vi "dsfsdfsd_Static1.vi"(8 "error in (no error)":errorcluster, 11 "dsfsdfsd in 1":refnum<class "dsfsdfsd.lvclass">) -> (0 "error out":errorcluster, 3 "dsfsdfsd  out":refnum<class "dsfsdfsd.lvclass">)   [LabVIEW 2013, in "dsfsdfsd.lvclass"]
uses:
  dsfsdfsd.lvclass
panel:
  in  "dsfsdfsd in 3":refnum<class "dsfsdfsd.lvclass">
  in  "dsfsdfsd in 2":refnum<class "dsfsdfsd.lvclass">
  out "Waveform Graph":dbl[](graph)
  in  "String":string
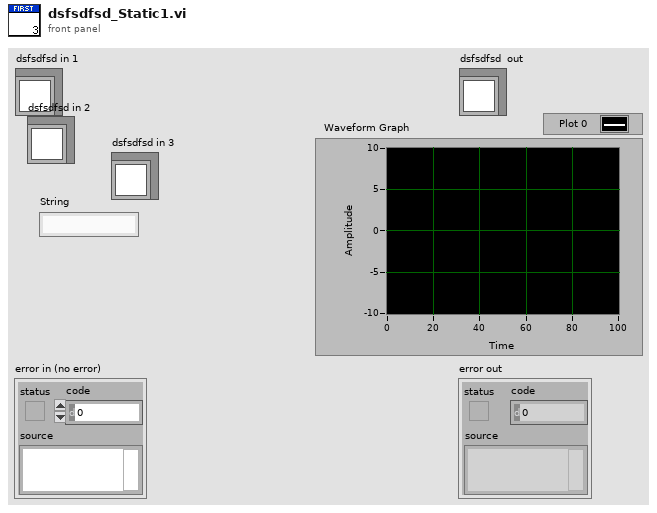
[diagram p1: front panel]
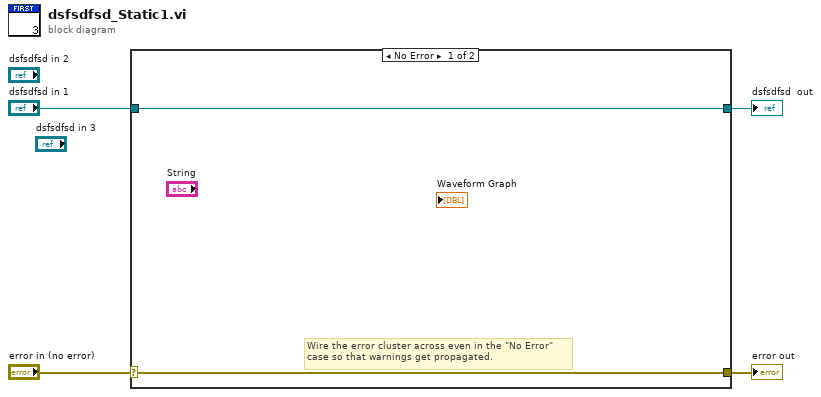
[diagram p0: block diagram]
diagram:
  n1 = case shown="No Error" "error in (no error)" {
    selector: "error in (no error)" -> [w5 w8]
    tunnel: [w5 w8] -> w3
    tunnel: [w6 w7] -> w1
    tunnel: "dsfsdfsd in 1" -> [w6 w7]
    frame No Error {
      # "Wire the error cluster across even in the \"No Error\"\ncase so that warnings get propagated."
    }
    frame Error {
    }
  }
  "error out" <- w3
  "dsfsdfsd  out" <- w1
